vi "Initial.vi"(8 "error in (no error)":errorcluster, 9 "Z":T2={"VISA resource name"="", "baud rate (9600)"=9600, "data bits (8)"=8, "parity (0:none)"=enum."None"} {"data bits (8)" min=5 max=8 step=1}, 10 "Y":T2={"VISA resource name"="", "baud rate (9600)"=9600, "data bits (8)"=8, "parity (0:none)"=enum."None"} {"data bits (8)" min=5 max=8 step=1}, 11 "X":T2={"VISA resource name"="", "baud rate (9600)"=9600, "data bits (8)"=8, "parity (0:none)"=enum."None"} {"data bits (8)" min=5 max=8 step=1}) -> (0 "error out":errorcluster, 3 "output cluster":T1)   [LabVIEW 2020, in "YP PowerControl.lvlib"]
uses:
  YP PowerControl.lvlib
  <vilib>/Instr/_visa.llb/VISA Configure Serial Port (Instr).vi
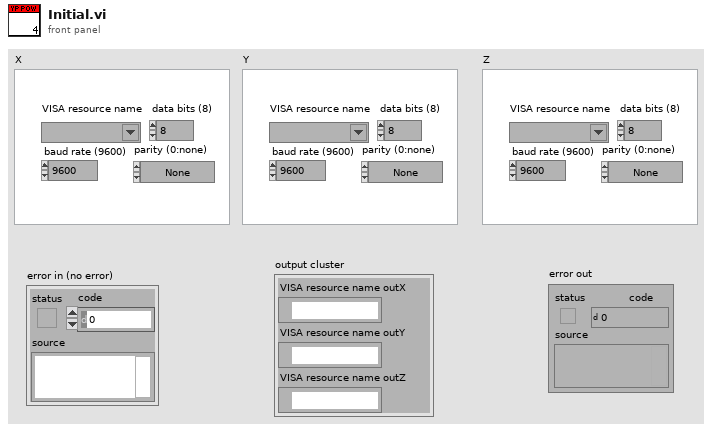
[diagram p1: front panel]
types:
  T1 = cluster{"VISA resource name outX":refnum<visa-resource-name>, "VISA resource name outY":refnum<visa-resource-name>, "VISA resource name outZ":refnum<visa-resource-name>}
  T2 = cluster{"VISA resource name":refnum<visa-resource-name>, "baud rate (9600)":u32, "data bits (8)":u16, "parity (0:none)":enum16{"None", "Odd", "Even", "Mark", "Space"}}
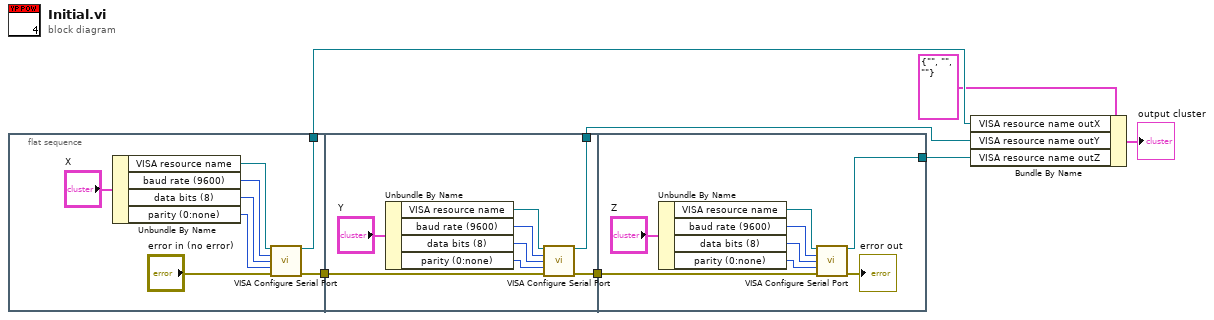
[diagram p0: block diagram]
diagram:
  n1 = flat-sequence {
    tunnel: [w9] -> w7
    tunnel: [w8] -> w1
    tunnel: [w18] -> w6
    tunnel: [w16] -> w2
    tunnel: w1 -> [w17]
    tunnel: [w26] -> w5
    tunnel: w2 -> [w25]
    frame #0 {
      n2 = Unbundle By Name("X") -> ("VISA resource name"=w13:refnum<visa-resource-name>, "baud rate (9600)"=w12:u32, "data bits (8)"=w11:u16, "parity (0:none)"=w10:enum16{"None", "Odd", "Even", "Mark", "Space"})
      n3 = call-poly "VISA Configure Serial Port"("VISA resource name"=w13, "baud rate (9600)"=w12, "data bits (8)"=w11, "parity (0:none)"=w10, "error in (no error)"="error in (no error)") -> ("VISA resource name out"=w9:refnum<visa-resource-name>, "error out"=w8:errorcluster)  [unwired: 9 in]
    }
    frame #1 {
      n4 = Unbundle By Name("Y") -> ("VISA resource name"=w19:refnum<visa-resource-name>, "baud rate (9600)"=w22:u32, "data bits (8)"=w21:u16, "parity (0:none)"=w20:enum16{"None", "Odd", "Even", "Mark", "Space"})
      n5 = call-poly "VISA Configure Serial Port"("VISA resource name"=w19, "baud rate (9600)"=w22, "data bits (8)"=w21, "parity (0:none)"=w20, "error in (no error)"=w17) -> ("VISA resource name out"=w18:refnum<visa-resource-name>, "error out"=w16:errorcluster)  [unwired: 9 in]
    }
    frame #2 {
      n6 = Unbundle By Name("Z") -> ("VISA resource name"=w30:refnum<visa-resource-name>, "baud rate (9600)"=w29:u32, "data bits (8)"=w28:u16, "parity (0:none)"=w27:enum16{"None", "Odd", "Even", "Mark", "Space"})
      n7 = call-poly "VISA Configure Serial Port"("VISA resource name"=w30, "baud rate (9600)"=w29, "data bits (8)"=w28, "parity (0:none)"=w27, "error in (no error)"=w25) -> ("VISA resource name out"=w26:refnum<visa-resource-name>, "error out"=→"error out":errorcluster)  [unwired: 9 in]
    }
  }
  n8 = Bundle By Name(cluster=T1 {"VISA resource name outX"="", "VISA resource name outY"="", "VISA resource name outZ"=""} ("rESULT"), "VISA resource name outX"=w7, "VISA resource name outY"=w6, "VISA resource name outZ"=w5) -> (→"output cluster":T1)
